vi "写入EPUB路径.vi"(8 "error in (no error)":errorcluster caption="错误输入（无错误）", 10 "EPUB路径":path, 11 "EPUB输入":refnum<class "EPUB.lvclass">) -> (0 "error out":errorcluster caption="错误输出", 3 "EPUB输出":refnum<class "EPUB.lvclass">)   [LabVIEW 2016, in "EPUB.lvclass"]
uses:
  EPUB.lvclass
  EPUB.lvclass/EPUB.ctl
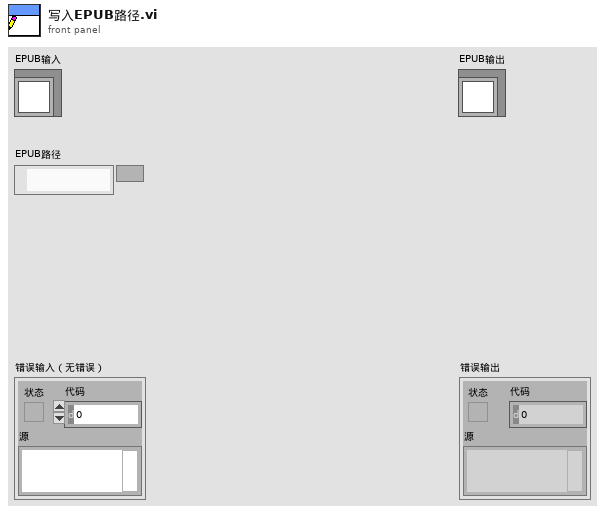
[diagram p1: front panel]
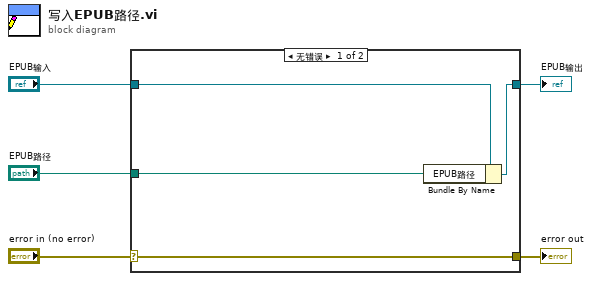
[diagram p0: block diagram]
diagram:
  n1 = case shown="无错误" "error in (no error)" {
    selector: "error in (no error)" -> [w9 w10]
    tunnel: [w9 w10] -> w4
    tunnel: [w7 w11] -> w2
    tunnel: "EPUB输入" -> [w8 w11]
    tunnel: "EPUB路径" -> [w6 _]
    frame No Error {
      n2 = Bundle By Name(cluster=w8, "EPUB路径"=w6) -> (w7:refnum<class "EPUB.lvclass">)
    }
    frame Error {
    }
  }
  "error out" <- w4
  "EPUB输出" <- w2
